vi "Read Polling Interval.vi"(8 "error in (no error)":errorcluster, 11 "CS++BaseActor in":refnum<class "CS++BaseActor.lvclass">) -> (0 "error out":errorcluster, 2 "Polling Interval":dbl[unit], 3 "CS++BaseActor out":refnum<class "CS++BaseActor.lvclass">)   [LabVIEW 2014, in "CS++BaseActor.lvlib" / "CS++BaseActor.lvclass"]
doc: "Intervall for periodic actions."
uses:
  CS++BaseActor.lvclass
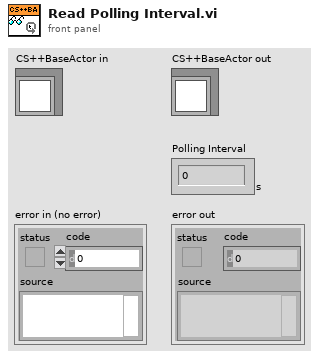
[diagram p1: front panel]
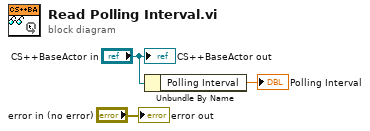
[diagram p0: block diagram]
diagram:
  n1 = Unbundle By Name("CS++BaseActor in") -> ("Polling Interval"=→"Polling Interval":dbl[unit])
  "error out" <- "error in (no error)"
  "CS++BaseActor out" <- "CS++BaseActor in"
